vi "S4GUI_003.vi"(7 "Tab ObsEng":enum32{"Obs", "CCD modes", "Guider", "Eng"}(tab)) -> ()   [LabVIEW 2018] (continued)
          tunnel: w8528 -> [w8553 w8580]
          tunnel: [w8544 w8568] -> w8526
          tunnel: w8525 -> [_ w8601]
          tunnel: w8524 -> [_ w8600]
          tunnel: w8523 -> [_ w8599]
          tunnel: w8522 -> [_ w8598]
          tunnel: w8521 -> [_ w8592]
          tunnel: w8514 -> [_ _]
          tunnel: w8512 -> [_ w8575]
          tunnel: w8511 -> [_ w8574]
          tunnel: w8510 -> [_ w8573]
          tunnel: w8509 -> [_ w8572]
          frame False {
            n3771 = call-dynamic "Read Acq_prevstate.vi"("error in (no error)"=w8550, "Acquisition in"=w8553) -> ("error out"=w8549:errorcluster, "Acq_prevstate"=w8551:u32, "Acquisition out"=w8552:refnum<class "Acquisition.lvclass">)  [unwired: 7 in]
            n3772 = call-dynamic "Write Acq_state.vi"("error in (no error)"=w8549, "Acq_state"=w8551, "Acquisition in"=w8552) -> ("error out"=w8540:errorcluster, "Acquisition out"=w8542:refnum<class "Acquisition.lvclass">)  [unwired: 7 in]
            n3773 = call-dynamic "Read enabled.vi"("error in (no error)"=w8540, "Server in"=w8542) -> ("error out"=w8539:errorcluster, "enabled"=w8536:bool, "Server out"=w8541:refnum<class "Acquisition.lvclass">)  [unwired: 7 in]
            n3774 = call-dynamic "Read Channel.vi"("error in (no error)"=w8539, "Acquisition in"=w8541) -> ("error out"=w8537:errorcluster, "Channel.lvclass"=w8538:refnum<class "Channel.lvclass">, "Acquisition out"=w8547:refnum<class "Acquisition.lvclass">)  [unwired: 7 in]
            n3775 = case shown="True" w8536 {
              tunnel: w8538 -> [w8555 w8565]
              tunnel: [w8555 w8563] -> w8546
              tunnel: w8537 -> [w8554 w8560]
              tunnel: [w8554 w8558] -> w8545
              frame False {
              }
              frame True {
                n3776 = call-dynamic "Read State Machine.vi"("error in (no error)"=w8560, "Device in"=w8565) -> ("error out"=w8556:errorcluster, "State Machine.lvclass"=w8557:refnum<class "State Machine.lvclass">, "Device out"=w8564:refnum<class "Channel.lvclass">)  [unwired: 7 in]
                n3777 = call "Next State.vi"("error in (no error)"=w8556, "New_State"=96, "State Machine in"=w8557) -> ("error out"=w8559:errorcluster, "State Machine out"=w8562:refnum<class "State Machine.lvclass">)  [unwired: 7 in]
                n3778 = call-dynamic "Write State Machine.vi"("error in (no error)"=w8559, "State Machine.lvclass"=w8562, "Device in"=w8564) -> ("error out"=w8558:errorcluster, "Device out"=w8563:refnum<class "Channel.lvclass">)  [unwired: 7 in]
              }
            }
            n3779 = call-dynamic "Write Channel.vi"("error in (no error)"=w8545, "Channel.lvclass"=w8546, "Acquisition in"=w8547) -> ("error out"=w8543:errorcluster, "Acquisition out"=w8544:refnum<class "Acquisition.lvclass">)  [unwired: 7 in]
          }
          frame True {
            # "obs type"
            # "suffix"
            # "object"
            n3780 = call "Read Instrument.lvclass.vi"("S4ACS_GUI in"=w8587) -> ("error out"=w8589:errorcluster, "Instrument.lvclass"=w8591:refnum<class "Instrument.lvclass">, "S4ACS_GUI out"=w8581:refnum<class "S4GUI.lvclass">)  [unwired: 8 in]
            n3781 = call "Read WPROT.vi"("error in (no error)"=w8589, "Instrument in"=w8591) -> ("error out"=w8588:errorcluster, "Opt_Selector.lvclass"=w8590:refnum<class "Opt_Selector.lvclass">)  [unwired: 7 in, 1 out]
            n3782 = call-dynamic "Read sequencia.vi"("error in (no error)"=w8588, "Opt_Selector in"=w8590) -> ()  [unwired: 7 in, 3 out]
            n3783 = case shown="Default" w8575 {
              tunnel: [u32 271 ("Obs_state") u32 251 ("Obs_state")] -> w8578
              tunnel: w8577 -> [w8626 w8637]
              tunnel: [w8625 w8637] -> w8576
              tunnel: w8574 -> [w8633 _]
              tunnel: w8573 -> [w8632 _]
              tunnel: w8572 -> [w8631 _]
              tunnel: w8581 -> [w8624 w8636]
              tunnel: [w8623 w8636] -> w8579
              frame "FOCUS" {
                n3784 = call-dynamic "Read TelFocus.lvclass.vi"("error in (no error)"=w8626, "S4GUI in"=w8624) -> ("error out"=w8628:errorcluster, "TelFocus.lvclass"=w8630:refnum<class "TelFocus.lvclass">, "S4GUI out"=w8634:refnum<class "S4GUI.lvclass">)  [unwired: 7 in]
                n3785 = call-dynamic "LoadParam.vi"("#steps"=w8631, "error in (no error)"=w8628, "step"=w8632, "init"=w8633, "TelFocus in"=w8630) -> ("error out"=w8627:errorcluster, "TelFocus out"=w8629:refnum<class "TelFocus.lvclass">)  [unwired: 5 in]
                n3786 = call-dynamic "Write TelFocus.lvclass.vi"("error in (no error)"=w8627, "TelFocus.lvclass"=w8629, "S4GUI in"=w8634) -> ("error out"=w8625:errorcluster, "S4GUI out"=w8623:refnum<class "S4GUI.lvclass">)  [unwired: 7 in]
              }
              frame Default {
              }
            }
            n3787 = property on="Start ch2" class="Bool"(error in=w8577, "DisabledEnum"=T12."Disabled and Grayed Out" ("Disabled")) -> ()  [unwired: 1 in, 2 out]
            n3788 = call-dynamic "Write Acq_state.vi"("error in (no error)"=w8576, "Acq_state"=w8578, "Acquisition in"=w8580) -> ("error out"=w8602:errorcluster, "Acquisition out"=w8603:refnum<class "Acquisition.lvclass">)  [unwired: 7 in]
            n3789 = call-dynamic "Read Channel.vi"("error in (no error)"=w8602, "Acquisition in"=w8603) -> ("error out"=w8604:errorcluster, "Channel.lvclass"=w8605:refnum<class "Channel.lvclass">, "Acquisition out"=w8609:refnum<class "Acquisition.lvclass">)  [unwired: 7 in]
            n3790 = call-dynamic "Read Interface.vi"("error in (no error)"=w8604, "Channel in"=w8605) -> ("error out"=w8621:errorcluster, "Interface.lvclass"=w8622:refnum<class "Interface.lvclass">, "Channel out"=w8620:refnum<class "Channel.lvclass">)  [unwired: 7 in]
            n3791 = call "Write Exposure Time.vi"("error in (no error)"=w8621, "Exposure Time"="Exptime ch2", "Interface in"=w8622) -> ("error out"=w8584:errorcluster, "Interface out"=w8586:refnum<class "Interface.lvclass">)  [unwired: 7 in]
            n3792 = case shown="Default" w8575 {
              tunnel: w8586 -> [w8640 w8645]
              tunnel: [w8640 w8644] -> w8585
              tunnel: w8584 -> [w8639 w8643]
              tunnel: [w8639 w8642] -> w8583
              tunnel: "Exptime ch2" -> [_ w8641]
              frame "ZERO" {
              }
              frame Default {
                n3793 = call-dynamic "Write prev ExpTime.vi"("error in (no error)"=w8643, "prev ExpTime"=w8641, "Interface in"=w8645) -> ("error out"=w8642:errorcluster, "Interface out"=w8644:refnum<class "Interface.lvclass">)  [unwired: 7 in]
              }
            }
            n3794 = call-dynamic "Write # Index.vi"("error in (no error)"=w8583, "# Index"="Index ch2", "Interface in"=w8585) -> ("error out"=w8618:errorcluster, "Interface out"=w8619:refnum<class "Interface.lvclass">)  [unwired: 7 in]
            n3795 = call-dynamic "Write Suffix.vi"("error in (no error)"=w8618, "Suffix"=w8601, "Interface in"=w8619) -> ("error out"=w8617:errorcluster, "Interface out"=w8616:refnum<class "Interface.lvclass">)  [unwired: 7 in]
            n3796 = call-dynamic "Write ObsType.vi"("error in (no error)"=w8617, "ObsType"=w8599, "Interface in"=w8616) -> ("error out"=w8614:errorcluster, "Interface out"=w8615:refnum<class "Interface.lvclass">)  [unwired: 7 in]
            n3797 = call-dynamic "Write Object.vi"("error in (no error)"=w8614, "Object"=w8598, "Interface in"=w8615) -> ("error out"=w8613:errorcluster, "Interface out"=w8612:refnum<class "Interface.lvclass">)  [unwired: 7 in]
            n3798 = call-dynamic "Write Comments.vi"("error in (no error)"=w8613, "Comments"=w8600, "Interface in"=w8612) -> ("error out"=w8610:errorcluster, "Interface out"=w8611:refnum<class "Interface.lvclass">)  [unwired: 7 in]
            n3799 = call-dynamic "Write DS9.vi"("error in (no error)"=w8610, "DS9"="F", "Interface in"=w8611) -> ("error out"=w8595:errorcluster, "Interface out"=w8597:refnum<class "Interface.lvclass">)  [unwired: 7 in]
            n3800 = call-dynamic "Write Observer.vi"("error in (no error)"=w8595, "Observer"=w8592, "Interface in"=w8597) -> ("error out"=w8594:errorcluster, "Interface out"=w8596:refnum<class "Interface.lvclass">)  [unwired: 7 in]
            n3801 = property on="Exposure Time ch2" class="Slide (strict)"("Scale.Maximum"="Exptime ch2", "Scale.Minimum"=0.0 ("Scale.Range:Minimum")) -> ()  [unwired: 2 in, 2 out]
            n3802 = call-dynamic "Write Interface.vi"("error in (no error)"=w8594, "Interface.lvclass"=w8596, "Channel in"=w8620) -> ("error out"=w8566:errorcluster, "Channel out"=w8567:refnum<class "Channel.lvclass">)  [unwired: 7 in]
            n3803 = call-dynamic "Write Channel.vi"("error in (no error)"=w8566, "Channel.lvclass"=w8567, "Acquisition in"=w8609) -> ("error out"=w8570:errorcluster, "Acquisition out"=w8571:refnum<class "Acquisition.lvclass">)  [unwired: 7 in]
            n3804 = call-dynamic "CalcCubeDuration.vi"("error in (no error)"=w8570, "Acquisition in"=w8571) -> ("error out"=w8569:errorcluster, "Acquisition out"=w8568:refnum<class "Acquisition.lvclass">)  [unwired: 8 in]
          }
        }
        n3805 = call "Write AcquisitionB.vi"("error in (no error)"=w8513, "Acquisition.lvclass"=w8526, "S4ACS_GUI in"=w8527) -> ("error out"=w8506:errorcluster, "S4ACS_GUI out"=w8507:refnum<class "S4GUI.lvclass">)  [unwired: 7 in]
        n3806 = call-dynamic "Write User Event.vi"("error in (no error)"=w8506, "User Event"="START ASYNC CH2", "S4GUI in"=w8507) -> ("error out"=w8504:errorcluster, "S4GUI out"=w8505:refnum<class "S4GUI.lvclass">)  [unwired: 7 in]
      }
      event "Start ch3": Value Change {
        n3807 = event-data() -> ()  [unwired: 1 in, 6 out]
        n3808 = call "Read Instrument.lvclass.vi"("error in (no error)"=w8658, "S4ACS_GUI in"=w8660) -> ("error out"=w8661:errorcluster, "Instrument.lvclass"=w8662:refnum<class "Instrument.lvclass">, "S4ACS_GUI out"=w8659:refnum<class "S4GUI.lvclass">)  [unwired: 7 in]
        n3809 = call-dynamic "Read mode.vi"("error in (no error)"=w8661, "Instrument in"=w8662) -> ("error out"=w8657:errorcluster, "mode"=w8656:bool)  [unwired: 7 in, 1 out]
        n3810 = call-dynamic "Read AcquisitionC.vi"("error in (no error)"=w8657, "S4ACS_GUI in"=w8659) -> ("error out"=w8674:errorcluster, "Acquisition.lvclass"=w8675:refnum<class "Acquisition.lvclass">, "S4ACS_GUI out"=w8677:refnum<class "S4GUI.lvclass">)  [unwired: 7 in]
        n3811 = call-dynamic "Read Acq_state.vi"("error in (no error)"=w8674, "Acquisition in"=w8675) -> ("error out"=w8671:errorcluster, "Acq_state"=w8673:u32, "Acquisition out"=w8670:refnum<class "Acquisition.lvclass">)  [unwired: 7 in]
        n3812 = Not Equal?(x=w8673, y=u32 400) -> (x != y?=w8676:bool)
        n3813 = case shown="True" w8676 {
          tunnel: w8677 -> [w8690 w8726]
          tunnel: [w8690 w8717] -> w8669
          tunnel: [w8685 w8709] -> w8655
          tunnel: w8671 -> [w8692 w8719]
          tunnel: w8670 -> [w8695 w8720]
          tunnel: [w8686 w8708] -> w8668
          tunnel: w8667 -> [_ w8739]
          tunnel: w8666 -> [_ w8738]
          tunnel: w8665 -> [_ w8737]
          tunnel: w8664 -> [_ w8736]
          tunnel: w8663 -> [_ w8731]
          tunnel: w8656 -> [_ _]
          tunnel: w8654 -> [_ w8715]
          tunnel: w8653 -> [_ w8714]
          tunnel: w8652 -> [_ w8713]
          tunnel: w8651 -> [_ w8712]
          frame False {
            n3814 = call-dynamic "Read Acq_prevstate.vi"("error in (no error)"=w8692, "Acquisition in"=w8695) -> ("error out"=w8691:errorcluster, "Acq_prevstate"=w8693:u32, "Acquisition out"=w8694:refnum<class "Acquisition.lvclass">)  [unwired: 7 in]
            n3815 = call-dynamic "Write Acq_state.vi"("error in (no error)"=w8691, "Acq_state"=w8693, "Acquisition in"=w8694) -> ("error out"=w8680:errorcluster, "Acquisition out"=w8682:refnum<class "Acquisition.lvclass">)  [unwired: 7 in]
            n3816 = call-dynamic "Read enabled.vi"("error in (no error)"=w8680, "Server in"=w8682) -> ("error out"=w8679:errorcluster, "enabled"=w8678:bool, "Server out"=w8681:refnum<class "Acquisition.lvclass">)  [unwired: 7 in]
            n3817 = call-dynamic "Read Channel.vi"("error in (no error)"=w8679, "Acquisition in"=w8681) -> ("error out"=w8683:errorcluster, "Channel.lvclass"=w8684:refnum<class "Channel.lvclass">, "Acquisition out"=w8688:refnum<class "Acquisition.lvclass">)  [unwired: 7 in]
            n3818 = case shown="True" w8678 {
              tunnel: w8684 -> [w8697 w8707]
              tunnel: [w8697 w8705] -> w8687
              tunnel: w8683 -> [w8696 w8702]
              tunnel: [w8696 w8700] -> w8689
              frame False {
              }
              frame True {
                n3819 = call-dynamic "Read State Machine.vi"("error in (no error)"=w8702, "Device in"=w8707) -> ("error out"=w8698:errorcluster, "State Machine.lvclass"=w8699:refnum<class "State Machine.lvclass">, "Device out"=w8706:refnum<class "Channel.lvclass">)  [unwired: 7 in]
                n3820 = call "Next State.vi"("error in (no error)"=w8698, "New_State"=96, "State Machine in"=w8699) -> ("error out"=w8701:errorcluster, "State Machine out"=w8704:refnum<class "State Machine.lvclass">)  [unwired: 7 in]
                n3821 = call-dynamic "Write State Machine.vi"("error in (no error)"=w8701, "State Machine.lvclass"=w8704, "Device in"=w8706) -> ("error out"=w8700:errorcluster, "Device out"=w8705:refnum<class "Channel.lvclass">)  [unwired: 7 in]
              }
            }
            n3822 = call-dynamic "Write Channel.vi"("error in (no error)"=w8689, "Channel.lvclass"=w8687, "Acquisition in"=w8688) -> ("error out"=w8685:errorcluster, "Acquisition out"=w8686:refnum<class "Acquisition.lvclass">)  [unwired: 7 in]
          }
          frame True {
            # "obs type"
            # "suffix"
            # "object"
            n3823 = call "Read Instrument.lvclass.vi"("S4ACS_GUI in"=w8726) -> ("error out"=w8728:errorcluster, "Instrument.lvclass"=w8730:refnum<class "Instrument.lvclass">, "S4ACS_GUI out"=w8718:refnum<class "S4GUI.lvclass">)  [unwired: 8 in]
            n3824 = call "Read WPROT.vi"("error in (no error)"=w8728, "Instrument in"=w8730) -> ("error out"=w8727:errorcluster, "Opt_Selector.lvclass"=w8729:refnum<class "Opt_Selector.lvclass">)  [unwired: 7 in, 1 out]
            n3825 = call-dynamic "Read sequencia.vi"("error in (no error)"=w8727, "Opt_Selector in"=w8729) -> ()  [unwired: 7 in, 3 out]
            n3826 = case shown="\"FOCUS\"" w8715 {
              tunnel: [u32 271 ("Obs_state") u32 251 ("Obs_state")] -> w8716
              tunnel: w8719 -> [w8767 w8778]
              tunnel: [w8766 w8778] -> _
              tunnel: w8714 -> [w8774 _]
              tunnel: w8713 -> [w8773 _]
              tunnel: w8712 -> [w8772 _]
              tunnel: w8718 -> [w8765 w8777]
              tunnel: [w8764 w8777] -> w8717
              frame "FOCUS" {
                n3827 = call-dynamic "Read TelFocus.lvclass.vi"("error in (no error)"=w8767, "S4GUI in"=w8765) -> ("error out"=w8769:errorcluster, "TelFocus.lvclass"=w8771:refnum<class "TelFocus.lvclass">, "S4GUI out"=w8775:refnum<class "S4GUI.lvclass">)  [unwired: 7 in]
                n3828 = call-dynamic "LoadParam.vi"("#steps"=w8772, "error in (no error)"=w8769, "step"=w8773, "init"=w8774, "TelFocus in"=w8771) -> ("error out"=w8768:errorcluster, "TelFocus out"=w8770:refnum<class "TelFocus.lvclass">)  [unwired: 5 in]
                n3829 = call-dynamic "Write TelFocus.lvclass.vi"("error in (no error)"=w8768, "TelFocus.lvclass"=w8770, "S4GUI in"=w8775) -> ("error out"=w8766:errorcluster, "S4GUI out"=w8764:refnum<class "S4GUI.lvclass">)  [unwired: 7 in]
              }
              frame Default {
              }
            }
            n3830 = call-dynamic "Write Acq_state.vi"("Acq_state"=w8716, "Acquisition in"=w8720) -> ("error out"=w8740:errorcluster, "Acquisition out"=w8741:refnum<class "Acquisition.lvclass">)  [unwired: 8 in]
            n3831 = call-dynamic "Read Channel.vi"("error in (no error)"=w8740, "Acquisition in"=w8741) -> ("error out"=w8742:errorcluster, "Channel.lvclass"=w8743:refnum<class "Channel.lvclass">, "Acquisition out"=w8750:refnum<class "Acquisition.lvclass">)  [unwired: 7 in]
            n3832 = property on="Start ch3" class="Bool"(error in=w8719, "DisabledEnum"=T12."Disabled and Grayed Out" ("Disabled")) -> ()  [unwired: 1 in, 2 out]
            n3833 = call-dynamic "Read Interface.vi"("error in (no error)"=w8742, "Channel in"=w8743) -> ("error out"=w8762:errorcluster, "Interface.lvclass"=w8763:refnum<class "Interface.lvclass">, "Channel out"=w8761:refnum<class "Channel.lvclass">)  [unwired: 7 in]
            n3834 = call "Write Exposure Time.vi"("error in (no error)"=w8762, "Exposure Time"="Exptime ch3", "Interface in"=w8763) -> ("error out"=w8723:errorcluster, "Interface out"=w8724:refnum<class "Interface.lvclass">)  [unwired: 7 in]
            n3835 = case shown="\"ZERO\"" w8715 {
              tunnel: [w8780 w8786] -> w8725
              tunnel: w8724 -> [w8780 w8785]
              tunnel: w8723 -> [w8781 w8784]
              tunnel: [w8781 w8783] -> w8722
              tunnel: "Exptime ch3" -> [_ w8782]
              frame "ZERO" {
              }
              frame Default {
                n3836 = call-dynamic "Write prev ExpTime.vi"("error in (no error)"=w8784, "prev ExpTime"=w8782, "Interface in"=w8785) -> ("error out"=w8783:errorcluster, "Interface out"=w8786:refnum<class "Interface.lvclass">)  [unwired: 7 in]
              }
            }
            n3837 = call-dynamic "Write # Index.vi"("error in (no error)"=w8722, "# Index"="Index ch3", "Interface in"=w8725) -> ("error out"=w8759:errorcluster, "Interface out"=w8760:refnum<class "Interface.lvclass">)  [unwired: 7 in]
            n3838 = call-dynamic "Write Suffix.vi"("error in (no error)"=w8759, "Suffix"=w8739, "Interface in"=w8760) -> ("error out"=w8758:errorcluster, "Interface out"=w8757:refnum<class "Interface.lvclass">)  [unwired: 7 in]
            n3839 = call-dynamic "Write ObsType.vi"("error in (no error)"=w8758, "ObsType"=w8736, "Interface in"=w8757) -> ("error out"=w8755:errorcluster, "Interface out"=w8756:refnum<class "Interface.lvclass">)  [unwired: 7 in]
            n3840 = call-dynamic "Write Object.vi"("error in (no error)"=w8755, "Object"=w8737, "Interface in"=w8756) -> ("error out"=w8754:errorcluster, "Interface out"=w8753:refnum<class "Interface.lvclass">)  [unwired: 7 in]
            n3841 = call-dynamic "Write Comments.vi"("error in (no error)"=w8754, "Comments"=w8738, "Interface in"=w8753) -> ("error out"=w8751:errorcluster, "Interface out"=w8752:refnum<class "Interface.lvclass">)  [unwired: 7 in]
            n3842 = call-dynamic "Write DS9.vi"("error in (no error)"=w8751, "DS9"="F", "Interface in"=w8752) -> ("error out"=w8733:errorcluster, "Interface out"=w8735:refnum<class "Interface.lvclass">)  [unwired: 7 in]
            n3843 = call-dynamic "Write Observer.vi"("error in (no error)"=w8733, "Observer"=w8731, "Interface in"=w8735) -> ("error out"=w8732:errorcluster, "Interface out"=w8734:refnum<class "Interface.lvclass">)  [unwired: 7 in]
            n3844 = call-dynamic "Write Interface.vi"("error in (no error)"=w8732, "Interface.lvclass"=w8734, "Channel in"=w8761) -> ("error out"=w8744:errorcluster, "Channel out"=w8745:refnum<class "Channel.lvclass">)  [unwired: 7 in]
            n3845 = property on="Exposure Time ch3" class="Slide (strict)"("Scale.Maximum"="Exptime ch3", "Scale.Minimum"=0.0 ("Scale.Range:Minimum")) -> ()  [unwired: 2 in, 2 out]
            n3846 = call-dynamic "Write Channel.vi"("error in (no error)"=w8744, "Channel.lvclass"=w8745, "Acquisition in"=w8750) -> ("error out"=w8710:errorcluster, "Acquisition out"=w8711:refnum<class "Acquisition.lvclass">)  [unwired: 7 in]
            n3847 = call-dynamic "CalcCubeDuration.vi"("error in (no error)"=w8710, "Acquisition in"=w8711) -> ("error out"=w8709:errorcluster, "Acquisition out"=w8708:refnum<class "Acquisition.lvclass">)  [unwired: 8 in]
          }
        }
        n3848 = call-dynamic "Write AcquisitionC.vi"("error in (no error)"=w8655, "Acquisition.lvclass"=w8668, "S4ACS_GUI in"=w8669) -> ("error out"=w8648:errorcluster, "S4ACS_GUI out"=w8649:refnum<class "S4GUI.lvclass">)  [unwired: 7 in]
        n3849 = call-dynamic "Write User Event.vi"("error in (no error)"=w8648, "User Event"="START ASYNC CH3", "S4GUI in"=w8649) -> ("error out"=w8647:errorcluster, "S4GUI out"=w8646:refnum<class "S4GUI.lvclass">)  [unwired: 7 in]
      }
      event "Start ch4": Value Change {
        n3850 = event-data() -> ()  [unwired: 1 in, 6 out]
        n3851 = call "Read Instrument.lvclass.vi"("error in (no error)"=w8801, "S4ACS_GUI in"=w8802) -> ("error out"=w8803:errorcluster, "Instrument.lvclass"=w8804:refnum<class "Instrument.lvclass">, "S4ACS_GUI out"=w8800:refnum<class "S4GUI.lvclass">)  [unwired: 7 in]
        n3852 = call-dynamic "Read mode.vi"("error in (no error)"=w8803, "Instrument in"=w8804) -> ("error out"=w8799:errorcluster, "mode"=w8798:bool)  [unwired: 7 in, 1 out]
        n3853 = call-dynamic "Read AcquisitionD.vi"("error in (no error)"=w8799, "S4ACS_GUI in"=w8800) -> ("error out"=w8815:errorcluster, "Acquisition.lvclass"=w8816:refnum<class "Acquisition.lvclass">, "S4ACS_GUI out"=w8818:refnum<class "S4GUI.lvclass">)  [unwired: 7 in]
        n3854 = call-dynamic "Read Acq_state.vi"("error in (no error)"=w8815, "Acquisition in"=w8816) -> ("error out"=w8812:errorcluster, "Acq_state"=w8814:u32, "Acquisition out"=w8811:refnum<class "Acquisition.lvclass">)  [unwired: 7 in]
        n3855 = Not Equal?(x=w8814, y=u32 400) -> (x != y?=w8817:bool)
        n3856 = case shown="True" w8817 {
          tunnel: w8818 -> [w8831 w8868]
          tunnel: [w8827 w8850] -> w8797
          tunnel: w8812 -> [w8833 w8860]
          tunnel: w8811 -> [w8836 w8861]
          tunnel: [w8826 w8849] -> w8810
          tunnel: w8809 -> [_ w8881]
          tunnel: w8808 -> [_ w8880]
          tunnel: w8807 -> [_ w8877]
          tunnel: w8806 -> [_ w8876]
          tunnel: w8805 -> [_ w8873]
          tunnel: w8798 -> [_ _]
          tunnel: [w8831 w8857] -> w8796
          tunnel: w8795 -> [_ w8856]
          tunnel: w8794 -> [_ w8855]
          tunnel: w8793 -> [_ w8854]
          tunnel: w8792 -> [_ w8853]
          frame False {
            n3857 = call-dynamic "Read Acq_prevstate.vi"("error in (no error)"=w8833, "Acquisition in"=w8836) -> ("error out"=w8832:errorcluster, "Acq_prevstate"=w8834:u32, "Acquisition out"=w8835:refnum<class "Acquisition.lvclass">)  [unwired: 7 in]
            n3858 = call-dynamic "Write Acq_state.vi"("error in (no error)"=w8832, "Acq_state"=w8834, "Acquisition in"=w8835) -> ("error out"=w8821:errorcluster, "Acquisition out"=w8825:refnum<class "Acquisition.lvclass">)  [unwired: 7 in]
            n3859 = call-dynamic "Read enabled.vi"("error in (no error)"=w8821, "Server in"=w8825) -> ("error out"=w8820:errorcluster, "enabled"=w8819:bool, "Server out"=w8824:refnum<class "Acquisition.lvclass">)  [unwired: 7 in]
            n3860 = call-dynamic "Read Channel.vi"("error in (no error)"=w8820, "Acquisition in"=w8824) -> ("error out"=w8822:errorcluster, "Channel.lvclass"=w8823:refnum<class "Channel.lvclass">, "Acquisition out"=w8829:refnum<class "Acquisition.lvclass">)  [unwired: 7 in]
            n3861 = case shown="True" w8819 {
              tunnel: w8823 -> [w8838 w8848]
              tunnel: [w8838 w8846] -> w8828
              tunnel: w8822 -> [w8837 w8843]
              tunnel: [w8837 w8841] -> w8830
              frame False {
              }
              frame True {
                n3862 = call-dynamic "Read State Machine.vi"("error in (no error)"=w8843, "Device in"=w8848) -> ("error out"=w8839:errorcluster, "State Machine.lvclass"=w8840:refnum<class "State Machine.lvclass">, "Device out"=w8847:refnum<class "Channel.lvclass">)  [unwired: 7 in]
                n3863 = call "Next State.vi"("error in (no error)"=w8839, "New_State"=96, "State Machine in"=w8840) -> ("error out"=w8842:errorcluster, "State Machine out"=w8845:refnum<class "State Machine.lvclass">)  [unwired: 7 in]
                n3864 = call-dynamic "Write State Machine.vi"("error in (no error)"=w8842, "State Machine.lvclass"=w8845, "Device in"=w8847) -> ("error out"=w8841:errorcluster, "Device out"=w8846:refnum<class "Channel.lvclass">)  [unwired: 7 in]
              }
            }
            n3865 = call-dynamic "Write Channel.vi"("error in (no error)"=w8830, "Channel.lvclass"=w8828, "Acquisition in"=w8829) -> ("error out"=w8827:errorcluster, "Acquisition out"=w8826:refnum<class "Acquisition.lvclass">)  [unwired: 7 in]
          }
          frame True {
            # "obs type"
            # "suffix"
            # "object"
            n3866 = call "Read Instrument.lvclass.vi"("S4ACS_GUI in"=w8868) -> ("error out"=w8870:errorcluster, "Instrument.lvclass"=w8872:refnum<class "Instrument.lvclass">, "S4ACS_GUI out"=w8858:refnum<class "S4GUI.lvclass">)  [unwired: 8 in]
            n3867 = call "Read WPROT.vi"("error in (no error)"=w8870, "Instrument in"=w8872) -> ("error out"=w8869:errorcluster, "Opt_Selector.lvclass"=w8871:refnum<class "Opt_Selector.lvclass">)  [unwired: 7 in, 1 out]
            n3868 = call-dynamic "Read sequencia.vi"("error in (no error)"=w8869, "Opt_Selector in"=w8871) -> ()  [unwired: 7 in, 3 out]
            n3869 = case shown="\"FOCUS\"" w8856 {
              tunnel: [u32 271 ("Obs_state") u32 251 ("Obs_state")] -> w8862
              tunnel: w8860 -> [w8909 w8920]
              tunnel: [w8908 w8920] -> w8859
              tunnel: w8855 -> [w8916 _]
              tunnel: w8854 -> [w8915 _]
              tunnel: w8853 -> [w8914 _]
              tunnel: w8858 -> [w8907 w8919]
              tunnel: [w8906 w8919] -> w8857
              frame "FOCUS" {
                n3870 = call-dynamic "Read TelFocus.lvclass.vi"("error in (no error)"=w8909, "S4GUI in"=w8907) -> ("error out"=w8911:errorcluster, "TelFocus.lvclass"=w8913:refnum<class "TelFocus.lvclass">, "S4GUI out"=w8917:refnum<class "S4GUI.lvclass">)  [unwired: 7 in]
                n3871 = call-dynamic "LoadParam.vi"("#steps"=w8914, "error in (no error)"=w8911, "step"=w8915, "init"=w8916, "TelFocus in"=w8913) -> ("error out"=w8910:errorcluster, "TelFocus out"=w8912:refnum<class "TelFocus.lvclass">)  [unwired: 5 in]
                n3872 = call-dynamic "Write TelFocus.lvclass.vi"("error in (no error)"=w8910, "TelFocus.lvclass"=w8912, "S4GUI in"=w8917) -> ("error out"=w8908:errorcluster, "S4GUI out"=w8906:refnum<class "S4GUI.lvclass">)  [unwired: 7 in]
              }
              frame Default {
              }
            }
            n3873 = call-dynamic "Write Acq_state.vi"("error in (no error)"=w8859, "Acq_state"=w8862, "Acquisition in"=w8861) -> ("error out"=w8882:errorcluster, "Acquisition out"=w8883:refnum<class "Acquisition.lvclass">)  [unwired: 7 in]
            n3874 = call-dynamic "Read Channel.vi"("error in (no error)"=w8882, "Acquisition in"=w8883) -> ("error out"=w8884:errorcluster, "Channel.lvclass"=w8885:refnum<class "Channel.lvclass">, "Acquisition out"=w8892:refnum<class "Acquisition.lvclass">)  [unwired: 7 in]
            n3875 = call-dynamic "Read Interface.vi"("error in (no error)"=w8884, "Channel in"=w8885) -> ("error out"=w8904:errorcluster, "Interface.lvclass"=w8905:refnum<class "Interface.lvclass">, "Channel out"=w8903:refnum<class "Channel.lvclass">)  [unwired: 7 in]
            n3876 = property on="Start ch4" class="Bool"(error in=w8860, "DisabledEnum"=T12."Disabled and Grayed Out" ("Disabled")) -> ()  [unwired: 1 in, 2 out]
            n3877 = call "Write Exposure Time.vi"("error in (no error)"=w8904, "Exposure Time"="Exptime ch4", "Interface in"=w8905) -> ("error out"=w8864:errorcluster, "Interface out"=w8867:refnum<class "Interface.lvclass">)  [unwired: 7 in]
            n3878 = case shown="\"ZERO\"" w8856 {
              tunnel: w8867 -> [w8923 w8928]
              tunnel: [w8923 w8927] -> w8866
              tunnel: [w8922 w8926] -> w8865
              tunnel: w8864 -> [w8922 w8925]
              tunnel: "Exptime ch4" -> [_ w8924]
              frame "ZERO" {
              }
              frame Default {
                n3879 = call-dynamic "Write prev ExpTime.vi"("error in (no error)"=w8925, "prev ExpTime"=w8924, "Interface in"=w8928) -> ("error out"=w8926:errorcluster, "Interface out"=w8927:refnum<class "Interface.lvclass">)  [unwired: 7 in]
              }
            }
            n3880 = call-dynamic "Write # Index.vi"("error in (no error)"=w8865, "# Index"="Index ch4", "Interface in"=w8866) -> ("error out"=w8901:errorcluster, "Interface out"=w8902:refnum<class "Interface.lvclass">)  [unwired: 7 in]
            n3881 = call-dynamic "Write Suffix.vi"("error in (no error)"=w8901, "Suffix"=w8881, "Interface in"=w8902) -> ("error out"=w8900:errorcluster, "Interface out"=w8899:refnum<class "Interface.lvclass">)  [unwired: 7 in]
            n3882 = call-dynamic "Write ObsType.vi"("error in (no error)"=w8900, "ObsType"=w8877, "Interface in"=w8899) -> ("error out"=w8897:errorcluster, "Interface out"=w8898:refnum<class "Interface.lvclass">)  [unwired: 7 in]
            n3883 = call-dynamic "Write Object.vi"("error in (no error)"=w8897, "Object"=w8876, "Interface in"=w8898) -> ("error out"=w8896:errorcluster, "Interface out"=w8895:refnum<class "Interface.lvclass">)  [unwired: 7 in]
            n3884 = call-dynamic "Write Comments.vi"("error in (no error)"=w8896, "Comments"=w8880, "Interface in"=w8895) -> ("error out"=w8893:errorcluster, "Interface out"=w8894:refnum<class "Interface.lvclass">)  [unwired: 7 in]
            n3885 = call-dynamic "Write DS9.vi"("error in (no error)"=w8893, "DS9"="F", "Interface in"=w8894) -> ("error out"=w8874:errorcluster, "Interface out"=w8875:refnum<class "Interface.lvclass">)  [unwired: 7 in]
            n3886 = call-dynamic "Write Observer.vi"("error in (no error)"=w8874, "Observer"=w8873, "Interface in"=w8875) -> ("error out"=w8878:errorcluster, "Interface out"=w8879:refnum<class "Interface.lvclass">)  [unwired: 7 in]
            n3887 = property on="Exposure Time ch4" class="Slide (strict)"("Scale.Maximum"="Exptime ch4", "Scale.Minimum"=0.0 ("Scale.Range:Minimum")) -> ()  [unwired: 2 in, 2 out]
            n3888 = call-dynamic "Write Interface.vi"("error in (no error)"=w8878, "Interface.lvclass"=w8879, "Channel in"=w8903) -> ("error out"=w8886:errorcluster, "Channel out"=w8887:refnum<class "Channel.lvclass">)  [unwired: 7 in]
            n3889 = call-dynamic "Write Channel.vi"("error in (no error)"=w8886, "Channel.lvclass"=w8887, "Acquisition in"=w8892) -> ("error out"=w8851:errorcluster, "Acquisition out"=w8852:refnum<class "Acquisition.lvclass">)  [unwired: 7 in]
            n3890 = call-dynamic "CalcCubeDuration.vi"("error in (no error)"=w8851, "Acquisition in"=w8852) -> ("error out"=w8850:errorcluster, "Acquisition out"=w8849:refnum<class "Acquisition.lvclass">)  [unwired: 8 in]
          }
        }
        n3891 = call-dynamic "Write AcquisitionD.vi"("error in (no error)"=w8797, "Acquisition.lvclass"=w8810, "S4ACS_GUI in"=w8796) -> ("error out"=w8788:errorcluster, "S4ACS_GUI out"=w8790:refnum<class "S4GUI.lvclass">)  [unwired: 7 in]
        n3892 = call-dynamic "Write User Event.vi"("error in (no error)"=w8788, "User Event"="START ASYNC CH4", "S4GUI in"=w8790) -> ("error out"=w8787:errorcluster, "S4GUI out"=w8789:refnum<class "S4GUI.lvclass">)  [unwired: 7 in]
      }
      event "Exptime ch1": Value Change {
        n3893 = event-data() -> ("NewVal"=w8933:dbl)  [unwired: 1 in]
        n3894 = call-dynamic "Read AcquisitionA.vi"("error in (no error)"=w8932, "S4ACS_GUI in"=w8931) -> ("error out"=w8947:errorcluster, "Acquisition.lvclass"=w8948:refnum<class "Acquisition.lvclass">, "S4ACS_GUI out"=w8945:refnum<class "S4GUI.lvclass">)  [unwired: 7 in]
        n3895 = call-dynamic "Read Channel.vi"("error in (no error)"=w8947, "Acquisition in"=w8948) -> ("error out"=w8936:errorcluster, "Channel.lvclass"=w8937:refnum<class "Channel.lvclass">, "Acquisition out"=w8938:refnum<class "Acquisition.lvclass">)  [unwired: 7 in]
        n3896 = call-dynamic "Read Interface.vi"("error in (no error)"=w8936, "Channel in"=w8937) -> ("error out"=w8942:errorcluster, "Interface.lvclass"=w8943:refnum<class "Interface.lvclass">, "Channel out"=w8941:refnum<class "Channel.lvclass">)  [unwired: 7 in]
        n3897 = call "Write Exposure Time.vi"("error in (no error)"=w8942, "Exposure Time"=w8933, "Interface in"=w8943) -> ("error out"=w8934:errorcluster, "Interface out"=w8935:refnum<class "Interface.lvclass">)  [unwired: 7 in]
        n3898 = call-dynamic "Write Interface.vi"("error in (no error)"=w8934, "Interface.lvclass"=w8935, "Channel in"=w8941) -> ("error out"=w8940:errorcluster, "Channel out"=w8939:refnum<class "Channel.lvclass">)  [unwired: 7 in]
        n3899 = call-dynamic "Write Channel.vi"("error in (no error)"=w8940, "Channel.lvclass"=w8939, "Acquisition in"=w8938) -> ("error out"=w8944:errorcluster, "Acquisition out"=w8946:refnum<class "Acquisition.lvclass">)  [unwired: 7 in]
        n3900 = call-dynamic "Write AcquisitionA.vi"("error in (no error)"=w8944, "Acquisition.lvclass"=w8946, "S4ACS_GUI in"=w8945) -> ("error out"=w8930:errorcluster, "S4ACS_GUI out"=w8929:refnum<class "S4GUI.lvclass">)  [unwired: 7 in]
      }
      event "Exptime ch2": Value Change {
        n3901 = event-data() -> ("NewVal"=w8953:dbl)  [unwired: 1 in]
        n3902 = call "Read AcquisitionB.vi"("error in (no error)"=w8952, "S4ACS_GUI in"=w8951) -> ("error out"=w8967:errorcluster, "Acquisition.lvclass"=w8968:refnum<class "Acquisition.lvclass">, "S4ACS_GUI out"=w8965:refnum<class "S4GUI.lvclass">)  [unwired: 7 in]
        n3903 = call-dynamic "Read Channel.vi"("error in (no error)"=w8967, "Acquisition in"=w8968) -> ("error out"=w8956:errorcluster, "Channel.lvclass"=w8957:refnum<class "Channel.lvclass">, "Acquisition out"=w8958:refnum<class "Acquisition.lvclass">)  [unwired: 7 in]
        n3904 = call-dynamic "Read Interface.vi"("error in (no error)"=w8956, "Channel in"=w8957) -> ("error out"=w8962:errorcluster, "Interface.lvclass"=w8963:refnum<class "Interface.lvclass">, "Channel out"=w8961:refnum<class "Channel.lvclass">)  [unwired: 7 in]
        n3905 = call "Write Exposure Time.vi"("error in (no error)"=w8962, "Exposure Time"=w8953, "Interface in"=w8963) -> ("error out"=w8954:errorcluster, "Interface out"=w8955:refnum<class "Interface.lvclass">)  [unwired: 7 in]
        n3906 = call-dynamic "Write Interface.vi"("error in (no error)"=w8954, "Interface.lvclass"=w8955, "Channel in"=w8961) -> ("error out"=w8960:errorcluster, "Channel out"=w8959:refnum<class "Channel.lvclass">)  [unwired: 7 in]
        n3907 = call-dynamic "Write Channel.vi"("error in (no error)"=w8960, "Channel.lvclass"=w8959, "Acquisition in"=w8958) -> ("error out"=w8964:errorcluster, "Acquisition out"=w8966:refnum<class "Acquisition.lvclass">)  [unwired: 7 in]
        n3908 = call "Write AcquisitionB.vi"("error in (no error)"=w8964, "Acquisition.lvclass"=w8966, "S4ACS_GUI in"=w8965) -> ("error out"=w8950:errorcluster, "S4ACS_GUI out"=w8949:refnum<class "S4GUI.lvclass">)  [unwired: 7 in]
      }
      event "Exptime ch3": Value Change {
        n3909 = event-data() -> ("NewVal"=w8973:dbl)  [unwired: 1 in]
        n3910 = call-dynamic "Read AcquisitionC.vi"("error in (no error)"=w8972, "S4ACS_GUI in"=w8971) -> ("error out"=w8987:errorcluster, "Acquisition.lvclass"=w8988:refnum<class "Acquisition.lvclass">, "S4ACS_GUI out"=w8985:refnum<class "S4GUI.lvclass">)  [unwired: 7 in]
        n3911 = call-dynamic "Read Channel.vi"("error in (no error)"=w8987, "Acquisition in"=w8988) -> ("error out"=w8976:errorcluster, "Channel.lvclass"=w8977:refnum<class "Channel.lvclass">, "Acquisition out"=w8978:refnum<class "Acquisition.lvclass">)  [unwired: 7 in]
        n3912 = call-dynamic "Read Interface.vi"("error in (no error)"=w8976, "Channel in"=w8977) -> ("error out"=w8982:errorcluster, "Interface.lvclass"=w8983:refnum<class "Interface.lvclass">, "Channel out"=w8981:refnum<class "Channel.lvclass">)  [unwired: 7 in]
        n3913 = call "Write Exposure Time.vi"("error in (no error)"=w8982, "Exposure Time"=w8973, "Interface in"=w8983) -> ("error out"=w8974:errorcluster, "Interface out"=w8975:refnum<class "Interface.lvclass">)  [unwired: 7 in]
        n3914 = call-dynamic "Write Interface.vi"("error in (no error)"=w8974, "Interface.lvclass"=w8975, "Channel in"=w8981) -> ("error out"=w8980:errorcluster, "Channel out"=w8979:refnum<class "Channel.lvclass">)  [unwired: 7 in]
        n3915 = call-dynamic "Write Channel.vi"("error in (no error)"=w8980, "Channel.lvclass"=w8979, "Acquisition in"=w8978) -> ("error out"=w8984:errorcluster, "Acquisition out"=w8986:refnum<class "Acquisition.lvclass">)  [unwired: 7 in]
        n3916 = call-dynamic "Write AcquisitionC.vi"("error in (no error)"=w8984, "Acquisition.lvclass"=w8986, "S4ACS_GUI in"=w8985) -> ("error out"=w8970:errorcluster, "S4ACS_GUI out"=w8969:refnum<class "S4GUI.lvclass">)  [unwired: 7 in]
      }
      event "Exptime ch4": Value Change {
        n3917 = event-data() -> ("NewVal"=w8993:dbl)  [unwired: 1 in]
        n3918 = call-dynamic "Read AcquisitionD.vi"("error in (no error)"=w8992, "S4ACS_GUI in"=w8991) -> ("error out"=w9007:errorcluster, "Acquisition.lvclass"=w9008:refnum<class "Acquisition.lvclass">, "S4ACS_GUI out"=w9005:refnum<class "S4GUI.lvclass">)  [unwired: 7 in]
        n3919 = call-dynamic "Read Channel.vi"("error in (no error)"=w9007, "Acquisition in"=w9008) -> ("error out"=w8996:errorcluster, "Channel.lvclass"=w8997:refnum<class "Channel.lvclass">, "Acquisition out"=w8998:refnum<class "Acquisition.lvclass">)  [unwired: 7 in]
        n3920 = call-dynamic "Read Interface.vi"("error in (no error)"=w8996, "Channel in"=w8997) -> ("error out"=w9002:errorcluster, "Interface.lvclass"=w9003:refnum<class "Interface.lvclass">, "Channel out"=w9001:refnum<class "Channel.lvclass">)  [unwired: 7 in]
        n3921 = call "Write Exposure Time.vi"("error in (no error)"=w9002, "Exposure Time"=w8993, "Interface in"=w9003) -> ("error out"=w8994:errorcluster, "Interface out"=w8995:refnum<class "Interface.lvclass">)  [unwired: 7 in]
        n3922 = call-dynamic "Write Interface.vi"("error in (no error)"=w8994, "Interface.lvclass"=w8995, "Channel in"=w9001) -> ("error out"=w9000:errorcluster, "Channel out"=w8999:refnum<class "Channel.lvclass">)  [unwired: 7 in]
        n3923 = call-dynamic "Write Channel.vi"("error in (no error)"=w9000, "Channel.lvclass"=w8999, "Acquisition in"=w8998) -> ("error out"=w9004:errorcluster, "Acquisition out"=w9006:refnum<class "Acquisition.lvclass">)  [unwired: 7 in]
        n3924 = call-dynamic "Write AcquisitionD.vi"("error in (no error)"=w9004, "Acquisition.lvclass"=w9006, "S4ACS_GUI in"=w9005) -> ("error out"=w8990:errorcluster, "S4ACS_GUI out"=w8989:refnum<class "S4GUI.lvclass">)  [unwired: 7 in]
      }
      event "Stop ch1": Value Change {
        n3925 = event-data() -> ()  [unwired: 1 in, 6 out]
        n3926 = disable-structure shown="Enabled" {
          disable-tunnel: w9012 -> [w9045 w9073]
          disable-tunnel: w9011 -> [w9043 w9067]
          disable-tunnel: [w9025 w9066] -> w9010
          disable-tunnel: [w9013 w9073] -> w9009
          frame Disabled {
            # "Para movimento \nda lamina retardadora"
            # "Restaura a última sequência de lâminas"
            n3927 = call-dynamic "Read AcquisitionA.vi"("error in (no error)"=w9043, "S4ACS_GUI in"=w9045) -> ("error out"=w9047:errorcluster, "Acquisition.lvclass"=w9046:refnum<class "Acquisition.lvclass">, "S4ACS_GUI out"=w9044:refnum<class "S4GUI.lvclass">)  [unwired: 7 in]
            n3928 = disable-structure shown="Enabled" {
              disable-tunnel: w9047 -> [w9052 w9063]
              disable-tunnel: w9046 -> [w9051 w9064]
              disable-tunnel: [w9049 w9064] -> w9041
              disable-tunnel: [w9048 w9063] -> w9040
              frame Disabled {
                # "Só precisa enviar comando STOP quando\no controle dos ciclos for feito pelo ACS."
                n3929 = call-dynamic "Read Channel.vi"("error in (no error)"=w9052, "Acquisition in"=w9051) -> ("error out"=w9054:errorcluster, "Channel.lvclass"=w9053:refnum<class "Channel.lvclass">, "Acquisition out"=w9060:refnum<class "Acquisition.lvclass">)  [unwired: 7 in]
                n3930 = call-dynamic "Read State Machine.vi"("error in (no error)"=w9054, "Device in"=w9053) -> ("error out"=w9056:errorcluster, "State Machine.lvclass"=w9055:refnum<class "State Machine.lvclass">, "Device out"=w9058:refnum<class "Channel.lvclass">)  [unwired: 7 in]
                n3931 = call "Next State.vi"("error in (no error)"=w9056, "New_State"=u32 70, "State Machine in"=w9055) -> ("error out"=w9059:errorcluster, "State Machine out"=w9057:refnum<class "State Machine.lvclass">)  [unwired: 7 in]
                n3932 = call-dynamic "Write State Machine.vi"("error in (no error)"=w9059, "State Machine.lvclass"=w9057, "Device in"=w9058) -> ("error out"=w9061:errorcluster, "Device out"=w9062:refnum<class "Channel.lvclass">)  [unwired: 7 in]
                n3933 = call-dynamic "Write Channel.vi"("error in (no error)"=w9061, "Channel.lvclass"=w9062, "Acquisition in"=w9060) -> ("error out"=w9048:errorcluster, "Acquisition out"=w9049:refnum<class "Acquisition.lvclass">)  [unwired: 7 in]
              }
              frame Enabled {
                # "Não precisa enviar comando STOP para o ACS\nenquanto o controle dos ciclos for feito pela GUI."
              }
            }
            n3934 = call-dynamic "Write Acq_state.vi"("error in (no error)"=w9040, "Acq_state"=u32 0, "Acquisition in"=w9041) -> ("error out"=w9039:errorcluster, "Acquisition out"=w9038:refnum<class "Acquisition.lvclass">)  [unwired: 7 in]
            n3935 = call-dynamic "Write AcquisitionA.vi"("error in (no error)"=w9039, "Acquisition.lvclass"=w9038, "S4ACS_GUI in"=w9044) -> ("error out"=w9026:errorcluster, "S4ACS_GUI out"=w9024:refnum<class "S4GUI.lvclass">)  [unwired: 7 in]
            n3936 = call "Read Instrument.lvclass.vi"("error in (no error)"=w9026, "S4ACS_GUI in"=w9024) -> ("error out"=w9033:errorcluster, "Instrument.lvclass"=w9036:refnum<class "Instrument.lvclass">, "S4ACS_GUI out"=w9037:refnum<class "S4GUI.lvclass">)  [unwired: 7 in]
            n3937 = call "Read WPROT.vi"("error in (no error)"=w9033, "Instrument in"=w9036) -> ("error out"=w9032:errorcluster, "Opt_Selector.lvclass"=w9034:refnum<class "Opt_Selector.lvclass">, "Instrument out"=w9035:refnum<class "Instrument.lvclass">)  [unwired: 7 in]
            n3938 = call-dynamic "Read sequencia_ant.vi"("error in (no error)"=w9032, "Opt_Selector in"=w9034) -> ("error out"=w9028:errorcluster, "sequencia_ant"=w9027:u16, "Opt_Selector out"=w9029:refnum<class "Opt_Selector.lvclass">)  [unwired: 7 in]
            n3939 = call-dynamic "Write sequencia.vi"("error in (no error)"=w9028, "sequencia"=w9027, "Opt_Selector in"=w9029) -> ("error out"=w9015:errorcluster, "Opt_Selector out"=w9018:refnum<class "Opt_Selector.lvclass">)  [unwired: 7 in]
            n3940 = call-dynamic "Read State Machine.vi"("error in (no error)"=w9015, "Device in"=w9018) -> ("error out"=w9020:errorcluster, "State Machine.lvclass"=w9023:refnum<class "State Machine.lvclass">, "Device out"=w9017:refnum<class "Opt_Selector.lvclass">)  [unwired: 7 in]
            n3941 = call "Next State.vi"("error in (no error)"=w9020, "New_State"=10, "State Machine in"=w9023) -> ("error out"=w9019:errorcluster, "State Machine out"=w9022:refnum<class "State Machine.lvclass">)  [unwired: 7 in]
            n3942 = call-dynamic "Write State Machine.vi"("error in (no error)"=w9019, "State Machine.lvclass"=w9022, "Device in"=w9017) -> ("error out"=w9014:errorcluster, "Device out"=w9016:refnum<class "Opt_Selector.lvclass">)  [unwired: 7 in]
            n3943 = call "Write WPROT.vi"("error in (no error)"=w9014, "Opt_Selector.lvclass"=w9016, "Instrument in"=w9035) -> ("error out"=w9031:errorcluster, "Instrument out"=w9030:refnum<class "Instrument.lvclass">)  [unwired: 7 in]
            n3944 = call "Write Instrument.lvclass.vi"("error in (no error)"=w9031, "Instrument.lvclass"=w9030, "S4ACS_GUI in"=w9037) -> ("error out"=w9025:errorcluster, "S4ACS_GUI out"=w9013:refnum<class "S4GUI.lvclass">)  [unwired: 7 in]
          }
          frame Enabled {
            w9069 = FALSE ("Wait Until Done")
            n3945 = call <vilib>:"Application Directory.vi"() -> ("Application Directory"=w9065:path)
            n3946 = Build Path(base path=w9065, name or relative path="MsgStop1.vi") -> (appended path=w9072:path)
            n3947 = Open VI Reference(vi path=w9072, error in (no error)=w9067) -> (vi reference=w9071:refnum<vi>, error out=w9070:errorcluster)  [unwired: 4 in]
            n3948 = invoke class="VI" method="Run VI"(reference=w9071, error in=w9070, "Wait until done"=w9069, "Auto Dispose Ref"=w9069) -> (error out=w9066:errorcluster)  [unwired: 1 in, 4 out]
          }
        }
      }
      event "Stop ch2": Value Change {
        n3949 = event-data() -> ()  [unwired: 1 in, 6 out]
        n3950 = disable-structure shown="Enabled" {
          disable-tunnel: w9077 -> [w9110 w9131]
          disable-tunnel: w9076 -> [w9108 w9133]
          disable-tunnel: [w9090 w9132] -> w9075
          disable-tunnel: [w9078 w9131] -> w9074
          frame Disabled {
            # "Para movimento \nda lamina retardadora"
            # "Restaura a última sequência de lâminas"
            n3951 = call "Read AcquisitionB.vi"("error in (no error)"=w9108, "S4ACS_GUI in"=w9110) -> ("error out"=w9112:errorcluster, "Acquisition.lvclass"=w9111:refnum<class "Acquisition.lvclass">, "S4ACS_GUI out"=w9109:refnum<class "S4GUI.lvclass">)  [unwired: 7 in]
            n3952 = disable-structure shown="Enabled" {
              disable-tunnel: w9112 -> [w9117 w9128]
              disable-tunnel: w9111 -> [w9116 w9129]
              disable-tunnel: [w9114 w9129] -> w9106
              disable-tunnel: [w9113 w9128] -> w9105
              frame Disabled {
                # "Só precisa enviar comando STOP quando\no controle dos ciclos for feito pelo ACS."
                n3953 = call-dynamic "Read Channel.vi"("error in (no error)"=w9117, "Acquisition in"=w9116) -> ("error out"=w9119:errorcluster, "Channel.lvclass"=w9118:refnum<class "Channel.lvclass">, "Acquisition out"=w9125:refnum<class "Acquisition.lvclass">)  [unwired: 7 in]
                n3954 = call-dynamic "Read State Machine.vi"("error in (no error)"=w9119, "Device in"=w9118) -> ("error out"=w9121:errorcluster, "State Machine.lvclass"=w9120:refnum<class "State Machine.lvclass">, "Device out"=w9123:refnum<class "Channel.lvclass">)  [unwired: 7 in]
                n3955 = call "Next State.vi"("error in (no error)"=w9121, "New_State"=u32 70, "State Machine in"=w9120) -> ("error out"=w9124:errorcluster, "State Machine out"=w9122:refnum<class "State Machine.lvclass">)  [unwired: 7 in]
                n3956 = call-dynamic "Write State Machine.vi"("error in (no error)"=w9124, "State Machine.lvclass"=w9122, "Device in"=w9123) -> ("error out"=w9126:errorcluster, "Device out"=w9127:refnum<class "Channel.lvclass">)  [unwired: 7 in]
                n3957 = call-dynamic "Write Channel.vi"("error in (no error)"=w9126, "Channel.lvclass"=w9127, "Acquisition in"=w9125) -> ("error out"=w9113:errorcluster, "Acquisition out"=w9114:refnum<class "Acquisition.lvclass">)  [unwired: 7 in]
              }
              frame Enabled {
                # "Não precisa enviar comando STOP para o ACS\nenquanto o controle dos ciclos for feito pela GUI."
              }
            }
            n3958 = call-dynamic "Write Acq_state.vi"("error in (no error)"=w9105, "Acq_state"=u32 0, "Acquisition in"=w9106) -> ("error out"=w9104:errorcluster, "Acquisition out"=w9103:refnum<class "Acquisition.lvclass">)  [unwired: 7 in]
            n3959 = call "Write AcquisitionB.vi"("error in (no error)"=w9104, "Acquisition.lvclass"=w9103, "S4ACS_GUI in"=w9109) -> ("error out"=w9091:errorcluster, "S4ACS_GUI out"=w9089:refnum<class "S4GUI.lvclass">)  [unwired: 7 in]
            n3960 = call "Read Instrument.lvclass.vi"("error in (no error)"=w9091, "S4ACS_GUI in"=w9089) -> ("error out"=w9098:errorcluster, "Instrument.lvclass"=w9101:refnum<class "Instrument.lvclass">, "S4ACS_GUI out"=w9102:refnum<class "S4GUI.lvclass">)  [unwired: 7 in]
            n3961 = call "Read WPROT.vi"("error in (no error)"=w9098, "Instrument in"=w9101) -> ("error out"=w9097:errorcluster, "Opt_Selector.lvclass"=w9099:refnum<class "Opt_Selector.lvclass">, "Instrument out"=w9100:refnum<class "Instrument.lvclass">)  [unwired: 7 in]
            n3962 = call-dynamic "Read sequencia_ant.vi"("error in (no error)"=w9097, "Opt_Selector in"=w9099) -> ("error out"=w9093:errorcluster, "sequencia_ant"=w9092:u16, "Opt_Selector out"=w9094:refnum<class "Opt_Selector.lvclass">)  [unwired: 7 in]
            n3963 = call-dynamic "Write sequencia.vi"("error in (no error)"=w9093, "sequencia"=w9092, "Opt_Selector in"=w9094) -> ("error out"=w9080:errorcluster, "Opt_Selector out"=w9083:refnum<class "Opt_Selector.lvclass">)  [unwired: 7 in]
            n3964 = call-dynamic "Read State Machine.vi"("error in (no error)"=w9080, "Device in"=w9083) -> ("error out"=w9085:errorcluster, "State Machine.lvclass"=w9088:refnum<class "State Machine.lvclass">, "Device out"=w9082:refnum<class "Opt_Selector.lvclass">)  [unwired: 7 in]
            n3965 = call "Next State.vi"("error in (no error)"=w9085, "New_State"=10, "State Machine in"=w9088) -> ("error out"=w9084:errorcluster, "State Machine out"=w9087:refnum<class "State Machine.lvclass">)  [unwired: 7 in]
            n3966 = call-dynamic "Write State Machine.vi"("error in (no error)"=w9084, "State Machine.lvclass"=w9087, "Device in"=w9082) -> ("error out"=w9079:errorcluster, "Device out"=w9081:refnum<class "Opt_Selector.lvclass">)  [unwired: 7 in]
            n3967 = call "Write WPROT.vi"("error in (no error)"=w9079, "Opt_Selector.lvclass"=w9081, "Instrument in"=w9100) -> ("error out"=w9096:errorcluster, "Instrument out"=w9095:refnum<class "Instrument.lvclass">)  [unwired: 7 in]
            n3968 = call "Write Instrument.lvclass.vi"("error in (no error)"=w9096, "Instrument.lvclass"=w9095, "S4ACS_GUI in"=w9102) -> ("error out"=w9090:errorcluster, "S4ACS_GUI out"=w9078:refnum<class "S4GUI.lvclass">)  [unwired: 7 in]
          }
          frame Enabled {
            w9135 = FALSE ("Wait Until Done")
            n3969 = call <vilib>:"Application Directory.vi"() -> ("Application Directory"=w9130:path)
            n3970 = Build Path(base path=w9130, name or relative path="MsgStop2.vi") -> (appended path=w9138:path)
            n3971 = Open VI Reference(vi path=w9138, error in (no error)=w9133) -> (vi reference=w9137:refnum<vi>, error out=w9136:errorcluster)  [unwired: 4 in]
            n3972 = invoke class="VI" method="Run VI"(reference=w9137, error in=w9136, "Wait until done"=w9135, "Auto Dispose Ref"=w9135) -> (error out=w9132:errorcluster)  [unwired: 1 in, 4 out]
          }
        }
      }
      event "Stop ch3": Value Change {
        n3973 = event-data() -> ()  [unwired: 1 in, 6 out]
        n3974 = disable-structure shown="Enabled" {
          disable-tunnel: w9142 -> [w9175 w9196]
          disable-tunnel: w9141 -> [w9173 w9198]
          disable-tunnel: [w9155 w9197] -> w9140
          disable-tunnel: [w9143 w9196] -> w9139
          frame Disabled {
            # "Para movimento \nda lamina retardadora"
            # "Restaura a última sequência de lâminas"
            n3975 = call-dynamic "Read AcquisitionC.vi"("error in (no error)"=w9173, "S4ACS_GUI in"=w9175) -> ("error out"=w9177:errorcluster, "Acquisition.lvclass"=w9176:refnum<class "Acquisition.lvclass">, "S4ACS_GUI out"=w9174:refnum<class "S4GUI.lvclass">)  [unwired: 7 in]
            n3976 = disable-structure shown="Enabled" {
              disable-tunnel: w9177 -> [w9182 w9193]
              disable-tunnel: w9176 -> [w9181 w9194]
              disable-tunnel: [w9179 w9194] -> w9171
              disable-tunnel: [w9178 w9193] -> w9170
              frame Disabled {
                # "Só precisa enviar comando STOP quando\no controle dos ciclos for feito pelo ACS."
